vi "Server.vi"   [LabVIEW 2024]
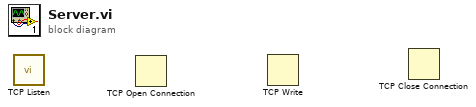
[diagram p0: block diagram]
diagram:
  n1 = call <vilib>:"TCP Listen.vi"() -> ()  [unwired: 7 in, 5 out]
  n2 = TCP Open Connection() -> ()  [unwired: 5 in, 2 out]
  n3 = TCP Write() -> ()  [unwired: 4 in, 3 out]
  n4 = TCP Close Connection() -> ()  [unwired: 3 in, 2 out]
